vi "Channel 2 Image Ring.vi"() -> ()   [LabVIEW 2016]
uses:
  <vilib>/vision/Image Controls.llb/IMAQ Image.ctl
panel:
  in  "Channel 2 Recon":T1
  in  "Channel 2 Ring Size":dbl
  in  "Channel 2 Index":dbl
  in  "Channel 2 Image":T1[](array[typedef])
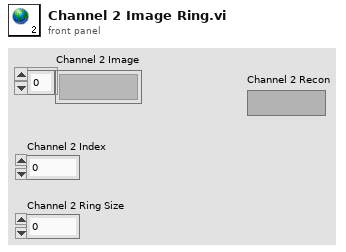
[diagram p1: front panel]
types:
  T1 = typedef "IMAQ Image.ctl" = refnum<image>
diagram:
